vi "写入configure.vi"(8 "error in (no error)":errorcluster caption="错误输入（无错误）", 10 "configure":T1={"IP"="", "PORT"="", "VISA resource name"="", "baud rate"=115200}, 11 "data_inter输入":refnum<class "data_inter.lvclass">) -> (0 "error out":errorcluster caption="错误输出", 3 "data_inter输出":refnum<class "data_inter.lvclass">)   [LabVIEW 2016, in "潮位站数据传输.lvlib" / "data_inter.lvclass"]
uses:
  data_inter.lvclass
  data_inter.lvclass/data_inter.ctl
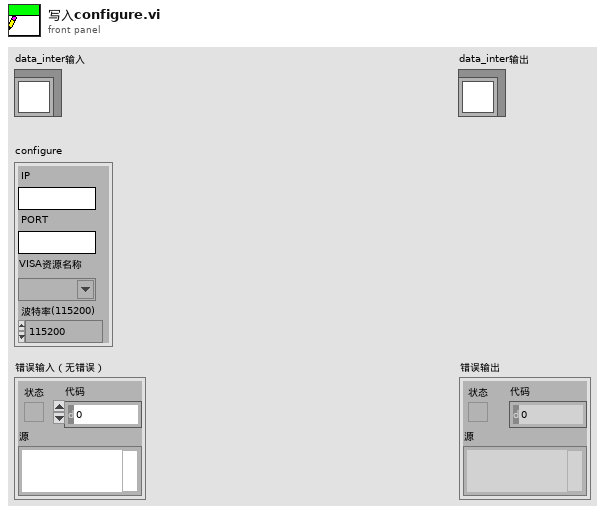
[diagram p1: front panel]
types:
  T1 = cluster{"IP":string, "PORT":string, "VISA resource name":refnum<visa-resource-name>, "baud rate":u32}
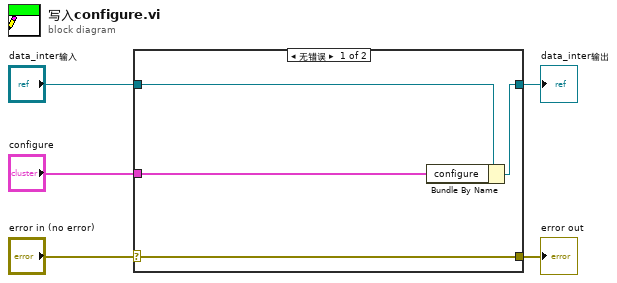
[diagram p0: block diagram]
diagram:
  n1 = case shown="无错误" "error in (no error)" {
    selector: "error in (no error)" -> [w9 w10]
    tunnel: [w9 w10] -> w4
    tunnel: [w7 w11] -> w2
    tunnel: "data_inter输入" -> [w8 w11]
    tunnel: "configure" -> [w6 _]
    frame No Error {
      n2 = Bundle By Name(cluster=w8, "configure"=w6) -> (w7:refnum<class "data_inter.lvclass">)
    }
    frame Error {
    }
  }
  "error out" <- w4
  "data_inter输出" <- w2
